vi "加标回收停止对话框.vi"() -> (2 "数组":bool[](array[boolean]), 3 "check？":bool)   [LabVIEW 2016, in "质控单元V1.lvlib"]
panel:
  in  "采配水":bool caption="启用"
  in  "取消":bool
  in  "确认":bool
  in  "CODCr":bool caption="启用"
  in  "CODMn":bool caption="启用"
  in  "总氮":bool caption="启用"
  in  "总磷":bool caption="启用"
  in  "氨氮":bool caption="启用"
  # "请选择要停止的参数"
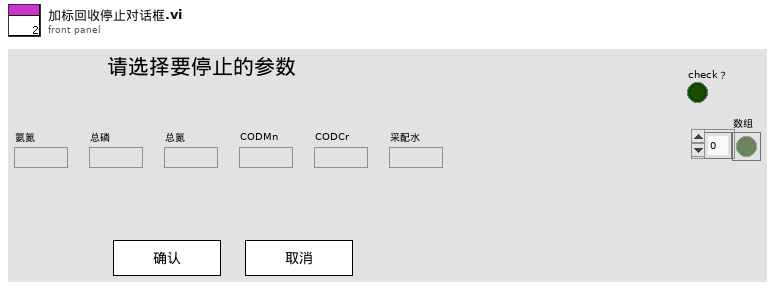
[diagram p1: front panel]
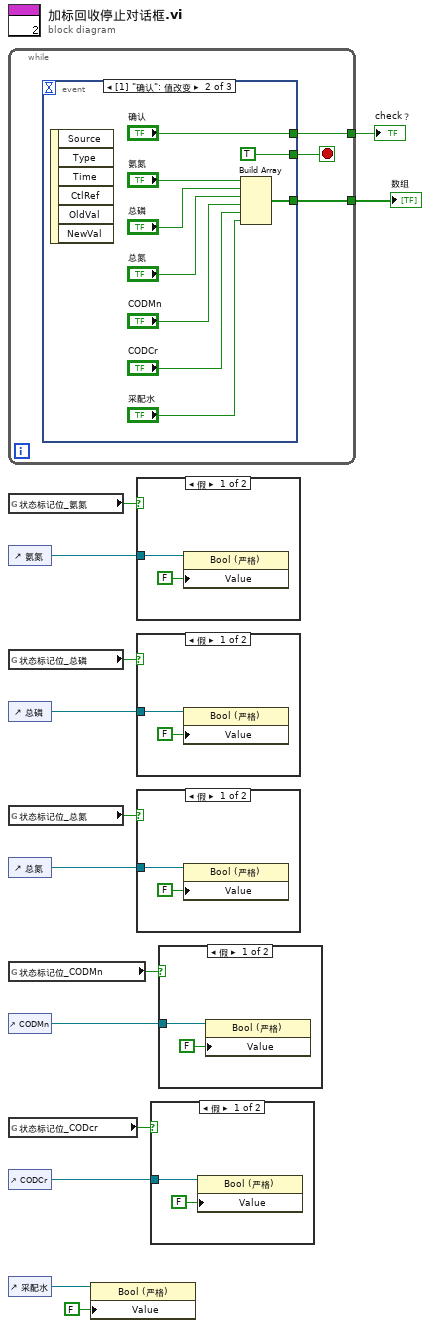
[diagram p0: block diagram]
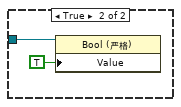
[diagram p2: hidden frame]
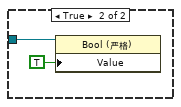
[diagram p3: hidden frame]
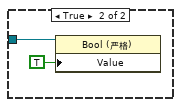
[diagram p4: hidden frame]
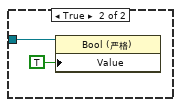
[diagram p5: hidden frame]
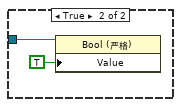
[diagram p6: hidden frame]
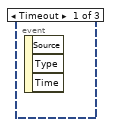
[diagram p7: hidden frame]
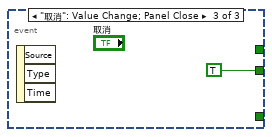
[diagram p8: hidden frame]
diagram:
  n1 = while {
    tunnel: [w16] -> w7
    tunnel: [w15] -> w6
    stop <- w17 stop-if-true
    n2 = event shown="[1] \"确认\": 值改变" {
      selector: _ -> [_ _ _]
      dyn-events: _ -> [_ _ _]
      timeout: _ -> [_ _ _]
      tunnel: [_ TRUE TRUE] -> w17
      tunnel: [_ w20 _] -> w16
      tunnel: [_ "确认" _] -> w15
      event Timeout {
        n3 = event-data() -> ()  [unwired: 1 in, 3 out]
      }
      event "确认": Value Change {
        n4 = event-data() -> ()  [unwired: 1 in, 6 out]
        n5 = Build Array("氨氮", "总磷", "总氮", "CODMn", "CODCr", "采配水") -> (w20:bool[])
      }
      event "取消": Value Change; Panel Close {
        n6 = event-data() -> ()  [unwired: 1 in, 3 out]
      }
    }
  }
  "数组" <- w7
  "check？" <- w6
  n7 = global read "ZK非断电保存全局变量.vi" "状态标记位_氨氮"() -> (w5:bool)
  n8 = control-ref of="氨氮"() -> (w14:refnum<vi>)
  n9 = global read "ZK非断电保存全局变量.vi" "状态标记位_总磷"() -> (w4:bool)
  n10 = control-ref of="总磷"() -> (w13:refnum<vi>)
  n11 = global read "ZK非断电保存全局变量.vi" "状态标记位_总氮"() -> (w3:bool)
  n12 = control-ref of="总氮"() -> (w12:refnum<vi>)
  n13 = global read "ZK非断电保存全局变量.vi" "状态标记位_CODMn"() -> (w2:bool)
  n14 = control-ref of="CODMn"() -> (w11:refnum<vi>)
  n15 = global read "ZK非断电保存全局变量.vi" "状态标记位_CODcr"() -> (w1:bool)
  n16 = control-ref of="CODCr"() -> (w10:refnum<vi>)
  n17 = control-ref of="采配水"() -> (w8:refnum<vi>)
  n18 = property class="Bool (严格)"(reference=w8, "Value"=FALSE ("值")) -> ()  [unwired: 1 in, 2 out]
  n19 = case shown="假" w5 {
    tunnel: w14 -> [w29 w31]
    frame False {
      n20 = property class="Bool (严格)"(reference=w29, "Value"=FALSE ("值")) -> ()  [unwired: 1 in, 2 out]
    }
    frame True {
      n21 = property class="Bool (严格)"(reference=w31, "Value"=TRUE ("值")) -> ()  [unwired: 1 in, 2 out]
    }
  }
  n22 = case shown="假" w4 {
    tunnel: w13 -> [w33 w35]
    frame False {
      n23 = property class="Bool (严格)"(reference=w33, "Value"=FALSE ("值")) -> ()  [unwired: 1 in, 2 out]
    }
    frame True {
      n24 = property class="Bool (严格)"(reference=w35, "Value"=TRUE ("值")) -> ()  [unwired: 1 in, 2 out]
    }
  }
  n25 = case shown="假" w3 {
    tunnel: w12 -> [w37 w39]
    frame False {
      n26 = property class="Bool (严格)"(reference=w37, "Value"=FALSE ("值")) -> ()  [unwired: 1 in, 2 out]
    }
    frame True {
      n27 = property class="Bool (严格)"(reference=w39, "Value"=TRUE ("值")) -> ()  [unwired: 1 in, 2 out]
    }
  }
  n28 = case shown="假" w1 {
    tunnel: w10 -> [w41 w43]
    frame False {
      n29 = property class="Bool (严格)"(reference=w41, "Value"=FALSE ("值")) -> ()  [unwired: 1 in, 2 out]
    }
    frame True {
      n30 = property class="Bool (严格)"(reference=w43, "Value"=TRUE ("值")) -> ()  [unwired: 1 in, 2 out]
    }
  }
  n31 = case shown="假" w2 {
    tunnel: w11 -> [w45 w47]
    frame False {
      n32 = property class="Bool (严格)"(reference=w45, "Value"=FALSE ("值")) -> ()  [unwired: 1 in, 2 out]
    }
    frame True {
      n33 = property class="Bool (严格)"(reference=w47, "Value"=TRUE ("值")) -> ()  [unwired: 1 in, 2 out]
    }
  }
